vi "Interface _Envio_Recepcion_Profe.vi"() -> ()   [LabVIEW 2017]
uses:
  <vilib>/Instr/_visa.llb/VISA Configure Serial Port (Instr).vi
panel:
  in  "Numeric":i32
  in  "Paro de emergencia":bool
  out "Number of bytes":u32
  out "Acelerómetro Motor 4":waveform(dbl)(graph)
  out "Acelerómetro Eje 2":waveform(dbl)(graph)
  out "Acelerómetro Eje 3":waveform(dbl)(graph)
  in  "Delay":u32
  out "Acelerómetro Carga 1":waveform(dbl)(graph)
  in  "Resetear Gráficos":bool
  out "Datos Crudos":string
  out "Status":bool
  in  "Puerto COM":refnum<visa-resource-name>
  out "String":string
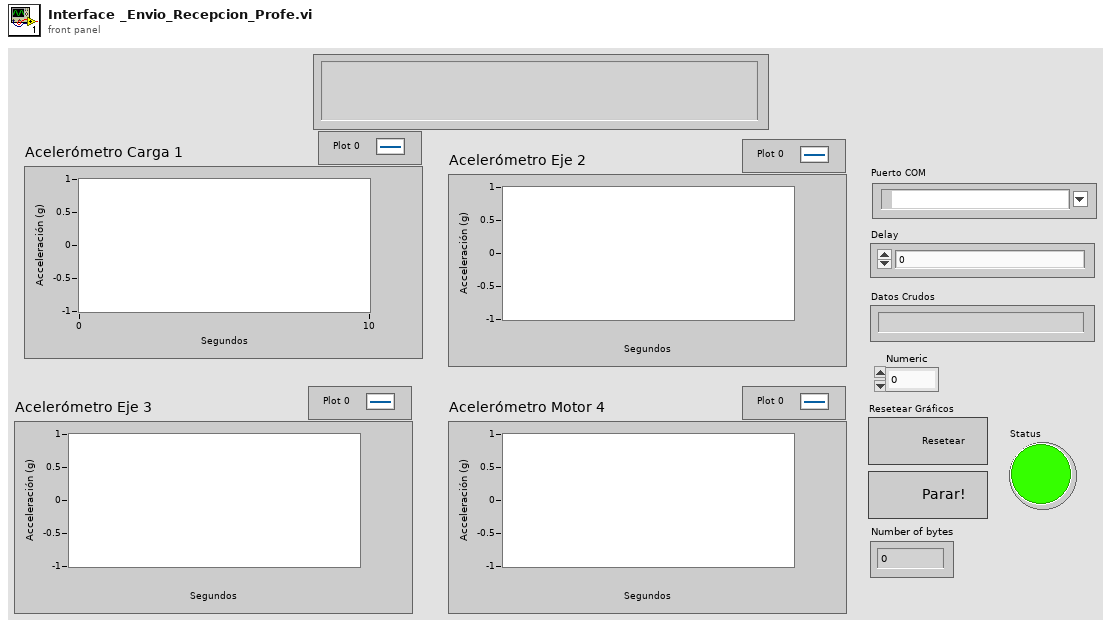
[diagram p1: front panel]
types:
  T1 = enum16{"Request", "Close", "Empty", "Decode", "Read", "Clear"}
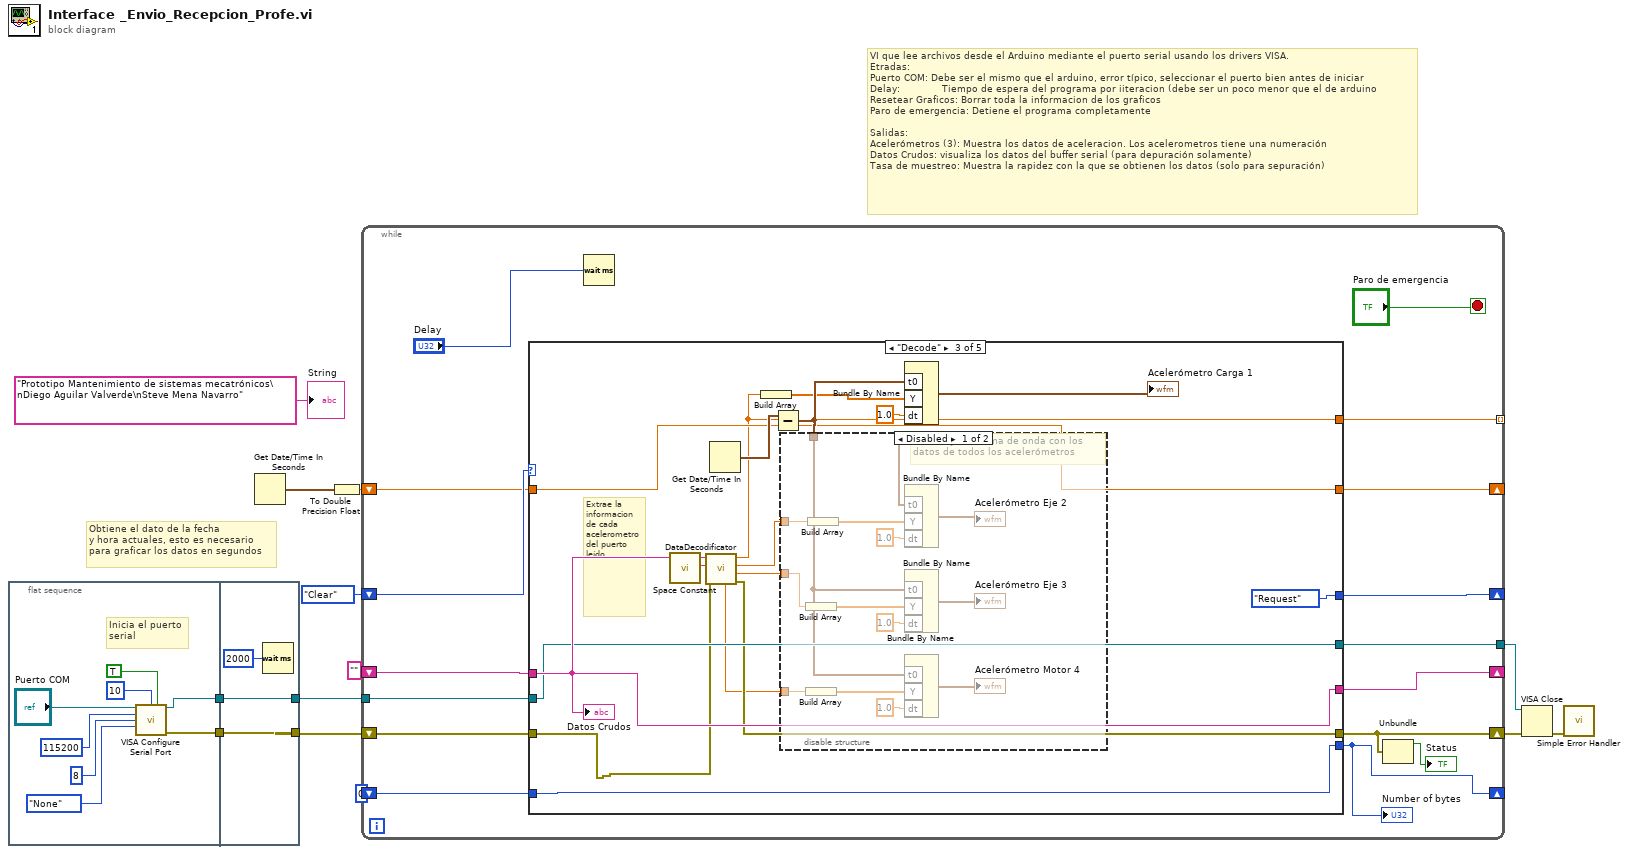
[diagram p0: block diagram]
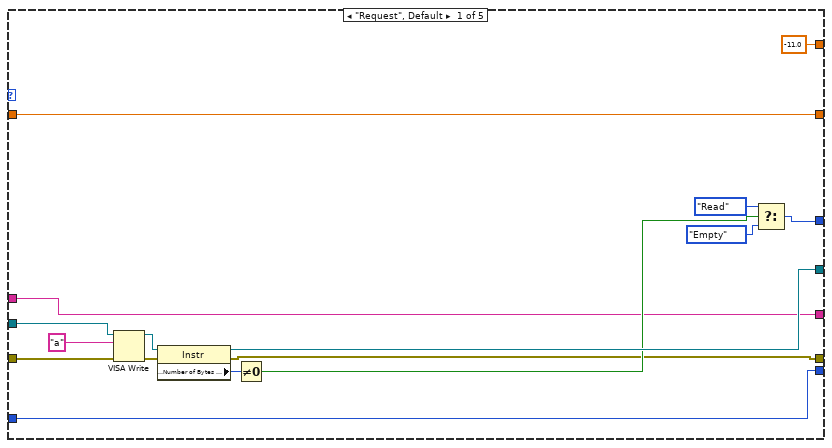
[diagram p2: hidden frame]
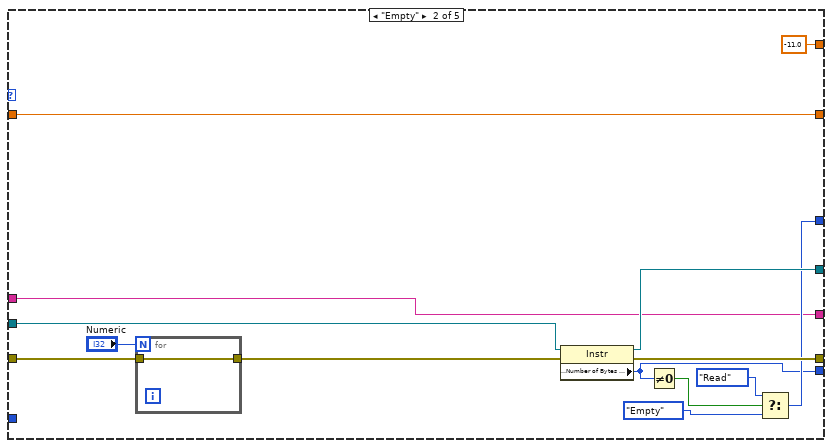
[diagram p3: hidden frame]
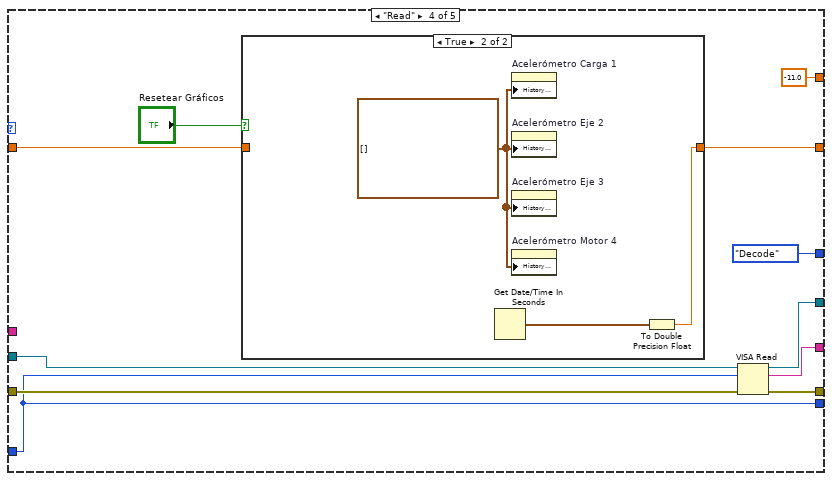
[diagram p5: hidden frame]
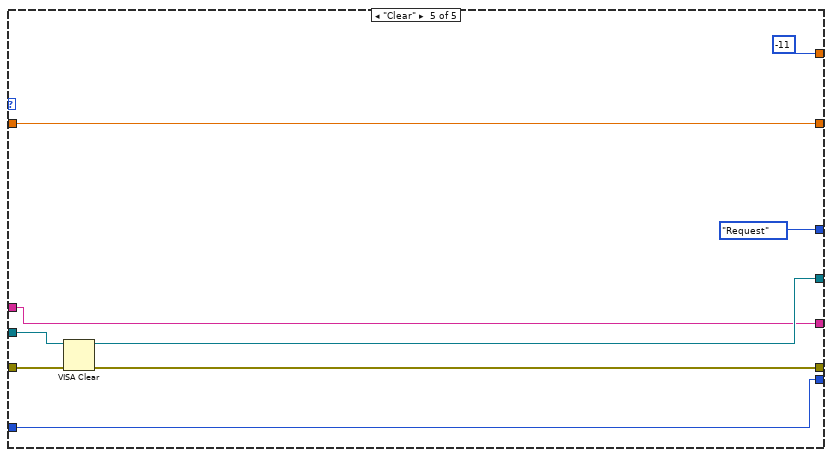
[diagram p7: hidden frame]
diagram:
  # "Obtiene el dato de la fecha \ny hora actuales, esto es necesario\npara graficar los datos en segundos"
  # "VI que lee archivos desde el Arduino mediante el puerto serial usando los drivers VISA.\nEtradas:\nPuerto COM: Debe ser el mismo que el arduino, error típico, seleccionar el puerto bien antes de iniciar\nDelay:              Tiempo de espera del programa por iiteracion (debe ser un poco menor que el de arduino\nResetear Graficos: Borrar toda la informacion de los graficos\nParo de emergencia: Detiene el programa completamente\n\nSalidas: \nAcelerómetros (3): Muestra los datos de aceleracion. Los acelerometros tiene una numeración\nDatos Crudos: visualiza los datos del buffer serial (para depuración solamente)\nTasa de muestreo: Muestra la rapidez con la que se obtienen los datos (solo para sepuración)"
  n1 = flat-sequence {
    tunnel: [w15] -> w2
    tunnel: [w14] -> w1
    tunnel: [w23] -> w9
    tunnel: [w24] -> w10
    tunnel: w2 -> [w24]
    tunnel: w1 -> [w23]
    frame #0 {
      # "Inicia el puerto\nserial"
      n2 = call-poly "VISA Configure Serial Port"("VISA resource name"="Puerto COM", "termination char\n(0xA = '\\n' = LF)"=u8 10 ("termination char\n(0xA = '\\n' = LF)"), "Enable Termination\nChar (T)"=TRUE ("Enable Termination\nChar (T)"), "baud rate (9600)"=u32 115200, "data bits (8)"=u16 8, "parity (0:none)"=enum16{"None", "Odd", "Even", "Mark", "Space"}."None") -> ("VISA resource name out"=w14:refnum<visa-resource-name>, "error out"=w15:errorcluster)  [unwired: 8 in]
    }
    frame #1 {
      n3 = Wait (ms)(milliseconds to wait=u32 2000) -> ()  [unwired: 1 out]
    }
  }
  n4 = Get Date/Time In Seconds() -> (seconds since 1Jan1904=w11:timestamp)
  n5 = To Double Precision Float(number=w11) -> (double precision float=w7:dbl)
  n6 = while {
    tunnel: w9 -> [w39]
    tunnel: [w38] -> w3
    shift-right: [w29] -> w5
    shift-left: w10 -> [w26]
    shift-right: [w37] -> _
    shift-left: T1."Clear" -> [w36]
    shift-right: [w27] -> _
    shift-left: u32 0 ("Bytes at Port") -> [w35]
    shift-right: [w34] -> _
    shift-left: "" ("read buffer") -> [w33]
    shift-right: [w30] -> _
    shift-left: w7 -> [w31]
    tunnel: [w25] -> _ mode=indexing
    stop <- "Paro de emergencia" stop-if-true
    n7 = case shown="\"Decode\"" w36 {
      tunnel: w26 -> [w46 w60 w74 w110 w125]
      tunnel: w39 -> [w55 w67 w80 w112 w124]
      tunnel: [w51 w66 w80 w111 w123] -> w38
      tunnel: [w42 w65 w78 w109 w122] -> w29
      tunnel: [w47 w64 T1."Request" T1."Decode" T1."Request"] -> w37
      tunnel: [w43 w63 w75 w108 w118] -> w27
      tunnel: w35 -> [w43 _ w75 w108 w118]
      tunnel: [w44 w62 w81 w107 w119] -> w34
      tunnel: w33 -> [w44 w62 w81 _ w119]
      tunnel: w31 -> [w45 w61 w82 w105 w120]
      tunnel: [w45 w61 w82 w103 w120] -> w30
      tunnel: [-11.0 ("Motor Accel 1") -11.0 ("Motor Accel 1") w72 -11.0 ("Motor Accel 1") -11] -> w25
      frame "Request", Default {
        n8 = VISA Write(VISA resource name=w55, write buffer="a", error in (no error)=w46) -> (VISA resource name out=w52:refnum<visa-resource-name>, error out=w53:errorcluster)  [unwired: 1 out]
        n9 = property class="Instr"(reference=w52, error in=w53) -> (reference out=w51:refnum<visa-resource-name>, error out=w42:errorcluster, "Serial Settings:Number of Bytes at Serial Port"=w54:u32)
        n10 = Not Equal To 0?(x=w54) -> (x != 0?=w50:bool)
        n11 = Select(t=T1."Read", s=w50, f=T1."Empty") -> (s? t:f=w47:T1)
      }
      frame "Empty" {
        n12 = for {
          N: "Numeric" -> [_]
          tunnel: w60 -> [w71]
          tunnel: [w71] -> w59
        }
        n13 = property class="Instr"(reference=w67, error in=w59) -> (reference out=w66:refnum<visa-resource-name>, error out=w65:errorcluster, "Serial Settings:Number of Bytes at Serial Port"=w63:u32)
        n14 = Not Equal To 0?(x=w63) -> (x != 0?=w70:bool)
        n15 = Select(t=T1."Read", s=w70, f=T1."Empty") -> (s? t:f=w64:T1)
      }
      frame "Decode" {
        # "Extrae la informacion de cada acelerometro del puerto leído"
        n16 = call <vilib>:"Space Constant.vi"() -> ("String"=w84:string)
        n17 = call "DataDecodificator.vi"(8:w74, "Separation Character"=w84, "Read Buffer"=w81) -> ("error out"=w78:errorcluster, "Bearing Accel 3"=w87:dbl, "Bearing Accel 2"=w86:dbl, "Motor Accel 1"=w72:dbl, "Load Accel 4"=w77:dbl)  [unwired: 4 in]
        n18 = Get Date/Time In Seconds() -> (seconds since 1Jan1904=w85:timestamp)
        n19 = Build Array(w72) -> (w73:dbl[])
        n20 = Subtract(x=w85, y=w82) -> (x-y=w88:timestamp)
        n21 = disable-structure shown="Disabled" {
          disable-tunnel: w88 -> [w101 _]
          disable-tunnel: w87 -> [w100 _]
          disable-tunnel: w86 -> [w99 _]
          disable-tunnel: w77 -> [w98 _]
          frame Disabled {
            # "Construye la forma de onda con los \ndatos de todos los acelerómetros"
            n22 = Build Array(w100) -> (w96:dbl[])
            n23 = Build Array(w98) -> (w97:dbl[])
            n24 = Build Array(w99) -> (w95:dbl[])
            n25 = Bundle By Name("t0"=w101, "Y"=w95, "dt"=1.0) -> (→"Acelerómetro Eje 2":waveform(dbl))  [unwired: 1 in]
            n26 = Bundle By Name("t0"=w101, "Y"=w96, "dt"=1.0) -> (→"Acelerómetro Eje 3":waveform(dbl))  [unwired: 1 in]
            n27 = Bundle By Name("t0"=w101, "Y"=w97, "dt"=1.0) -> (→"Acelerómetro Motor 4":waveform(dbl))  [unwired: 1 in]
          }
          frame Enabled {
          }
        }
        n28 = Bundle By Name("t0"=w88, "Y"=w73, "dt"=1.0) -> (→"Acelerómetro Carga 1":waveform(dbl))  [unwired: 1 in]
        "Datos Crudos" <- w81
      }
      frame "Read" {
        n29 = case shown="True" "Resetear Gráficos" {
          tunnel: w105 -> [w113 _]
          tunnel: [w113 w115] -> w103
          frame False {
          }
          frame True {
            w114 = waveform(dbl)[] [] ("History Data")
            n30 = Get Date/Time In Seconds() -> (seconds since 1Jan1904=w116:timestamp)
            n31 = property on="Acelerómetro Carga 1" class="WFChart (strict)"("History Data"=w114) -> ()  [unwired: 2 in, 2 out]
            n32 = property on="Acelerómetro Eje 2" class="WFChart (strict)"("History Data"=w114) -> ()  [unwired: 2 in, 2 out]
            n33 = property on="Acelerómetro Eje 3" class="WFChart (strict)"("History Data"=w114) -> ()  [unwired: 2 in, 2 out]
            n34 = property on="Acelerómetro Motor 4" class="WFChart (strict)"("History Data"=w114) -> ()  [unwired: 2 in, 2 out]
            n35 = To Double Precision Float(number=w116) -> (double precision float=w115:dbl)
          }
        }
        n36 = VISA Read(VISA resource name=w112, byte count=w108, error in (no error)=w110) -> (VISA resource name out=w111:refnum<visa-resource-name>, read buffer=w107:string, error out=w109:errorcluster)  [unwired: 1 out]
      }
      frame "Clear" {
        n37 = VISA Clear(VISA resource name=w124, error in (no error)=w125) -> (VISA resource name out=w123:refnum<visa-resource-name>, error out=w122:errorcluster)
      }
    }
    "Number of bytes" <- w27
    n38 = Wait (ms)(milliseconds to wait="Delay") -> ()  [unwired: 1 out]
    n39 = Unbundle(w29) -> ("status"=→"Status":bool)  [unwired: 2 out]
  }
  n40 = VISA Close(VISA resource name=w3, error in (no error)=w5) -> (error out=w12:errorcluster)
  n41 = call <vilib>:"Simple Error Handler.vi"("error in (no error)"=w12) -> ()  [unwired: 4 in, 5 out]
  "String" <- "Prototipo Mantenimiento de sistemas mecatrónicos\nDiego Aguilar Valverde\nSteve Mena Navarro"
